vi "SimulatoreStep.vi"() -> ()   [LabVIEW 2019]
doc: "Simulatore Step dei Test:\n\n1. Seleziona la postazione con la data di partenza (opzionale)\n2. Seleziona il Test che vuoi eseguire\n3. Avvia la simulazione e verifica il successo degli Step"
uses:
  ByteGSAPIBase.lvclass
  TypeDef/StepSimulationInfo.ctl
  TypeDef/ProcessStatus.ctl
  TypeDef/SimulatoreStates.ctl
  TypeDef/Step.ctl
  TypeDef/Asset.ctl
  TypeDef/Test.ctl
  <vilib>/numeric/Random Number (Range) U64.vi
  <vilib>/numeric/sub_Random U32.vi
panel:
  out "Status Control":T2={"Cluster"={"Active"=FALSE, "Process"="Acquisizione Dati"}, "Cluster 2"={"Active"=FALSE, "Process"="Upload Dati"}, "Cluster 3"={"Active"=FALSE, "Process"="Upload Completato"}}
  out "Waveform Chart":cluster{"Time Elapsed":dbl, dbl}(graph)
  out "Step Info List":T3[](array[typedef])=[{"info"="Descrizione:\nMeasure T0\nMIN - MAX: 23 - 18", "Value"=0.0, "Outcome"="", "Tempo"=0.0, "id"=0.0}, {"info"="Descrizione:\nSet Nominsl Torque\nMIN - MAX: 1 - -1", "Value"=0.0, "Outcome"="", "Tempo"=0.0, "id"=0.0}, {"info"="Descrizione:\nVibrazione X,Y,Z\nMIN - MAX: 0 - 0", "Value"=0.0, "Outcome"="", "Tempo"=0.0, "id"=0.0}, {"info"="Descrizione:\nPlace Motor on the bench. Plug wires on terminal block.\nMIN - MAX: 0 - 0", "Value"=0.0, "Outcome"="", "Tempo"=0.0, "id"=0.0}, {"info"="Descrizione:\nMeasure R01\nMIN - MAX: 0 - 0", "Value"=0.0, "Outcome"="", "Tempo"=0.0, "id"=0.0}, {"info"="Descrizione:\nMeasure R02\nMIN - MAX: 0 - 0", "Value"=0.0, "Outcome"="", "Tempo"=0.0, "id"=0.0}]
  in  "Step simulation":bool
  out "Infos":string
  in  "Inizia Test":bool
  in  "Seleziona Test":i32(ring) items=["Test Endurance"=36, "Test su Statore H100 dia 65"=31, "Test su Statore H100 dia 65"=29, "Test Endurance"=34, "Test su Statore H100 dia 65"=30, "Effettuare prova sul banco Labview su campione ABC"=40, "Test su Statore H100 dia 65"=28, "Test su Statore H100 dia 65"=32, "Richiesta prova 1"=7, "Test Endurance"=35, "Richiesta prova 1"=5, "Richiesta prova 1"=6, "Test su Statore H100 dia 65"=27, "Test doppio carico per freni 50Nm/12rpm"=24]
  in  "ByteGSAPIBase in":refnum<class "ByteGSAPIBase.lvclass">
  in  "Exit":bool
  in  "Home":bool
  in  "Ottieni Test Per Postazione":bool
  in  "Data Partenza":timestamp format="%<%x>T"
  in  "Postazione":enum16{"POST 1"}(ring)
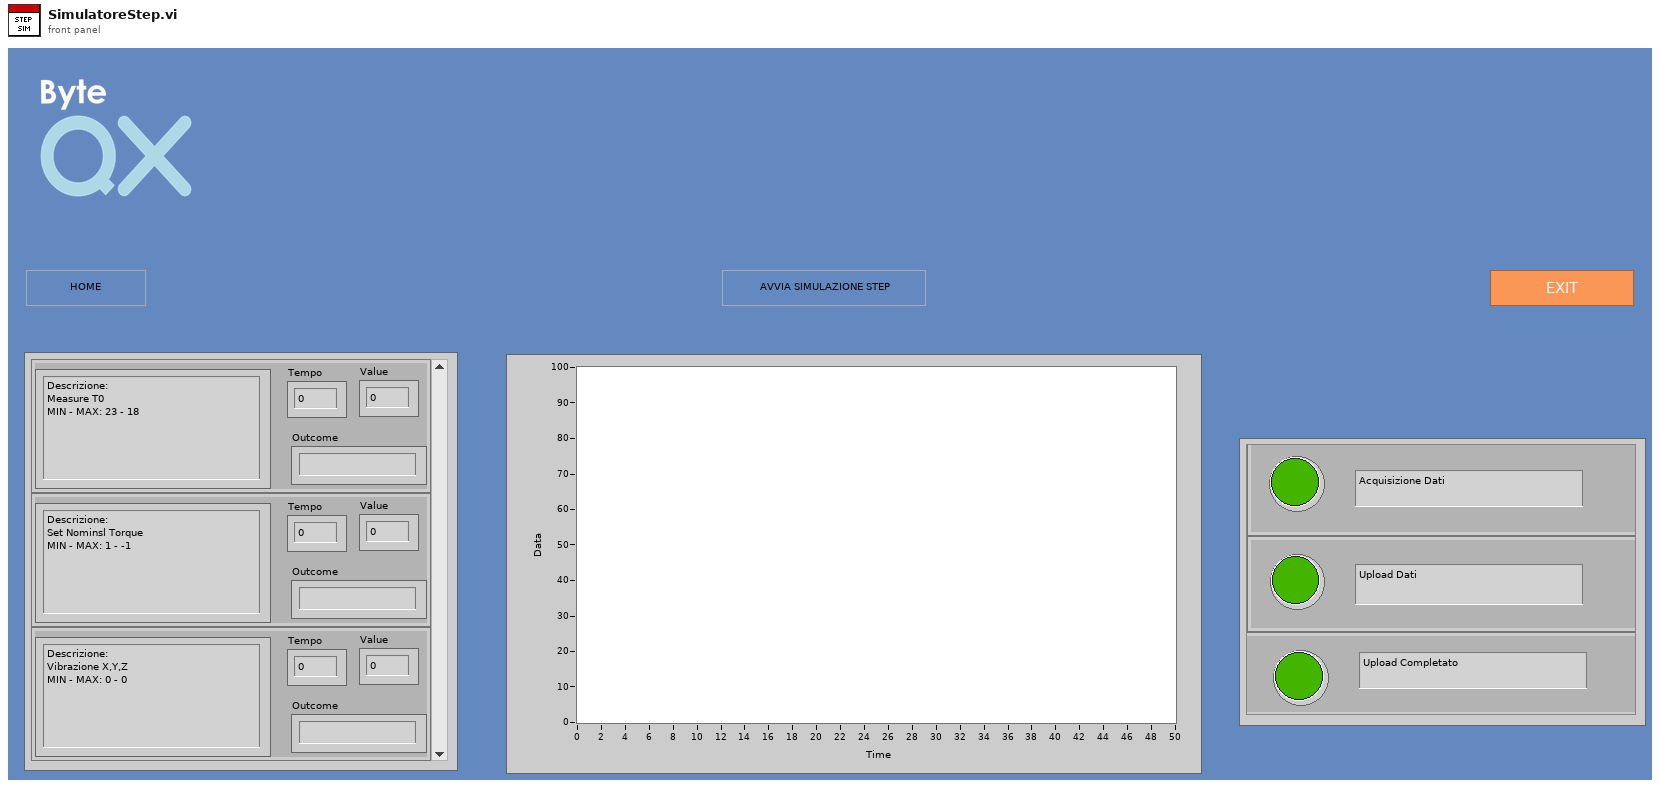
[diagram p1: front panel]
types:
  T1 = typedef "ProcessStatus.ctl" = cluster{"Active":bool, "Process":string}
  T2 = cluster{"Cluster":T1, "Cluster 2":T1, "Cluster 3":T1}
  T3 = typedef "StepSimulationInfo.ctl" = cluster{"info":string, "Value":dbl, "Outcome":string, "Tempo":dbl, "id":dbl}
  T4 = typedef "SimulatoreStates.ctl" = enum16{"Initialize", "Idle", "GetLimsTestsForBench", "GetLimsTestSteps", "Simulation Start", "WaitForLigths"}
  T5 = typedef "ByteGSWebAPI.lvlib/ByteGSAPIBase.lvclass/Test.ctl" = cluster{"titolo":string, "descrizione":string, "statoprova":string, "assets":T6[], "id":i32, "data_apertura_prova":timestamp}
  T6 = typedef "ByteGSWebAPI.lvlib/ByteGSAPIBase.lvclass/Asset.ctl" = cluster{"descrizione":string, "slug":string, "id":i32}
  T7 = typedef "ByteGSWebAPI.lvlib/ByteGSAPIBase.lvclass/Step.ctl" = cluster{"id":i32, "descrizione":string, "prova":string, "assets":T6[], "criterio_accettazione":string, "valore_criterio_accettazione_max":dbl, "valore_criterio_accettazione_min":dbl, "udm_criterio_accettazione":string, "duration_prova":string, "udm_duration_prova":string, "valore_prova":dbl, "ordine":i32, "user":i32, "link_automation":string, "instruction_automation":string, "data_completamento_checklist":timestamp, "outcome":bool}
  T8 = cluster{"ByteGSAPIBase in":refnum<class "ByteGSAPIBase.lvclass">, "Array dei Test":T5[], "Steps Array":T7[], "Step Info List":T3[], "index":i32, "Previus":T4, "Infos":string, "State":T4, "Status Control":cluster{"Cluster":T1, "Cluster 2":T1, "Cluster 3":T1}, "light position":i32}
  T9 = cluster{"Postazione":refnum<vi>, "Data Partenza":refnum<vi>, "Ottieni Test Per Postazione":refnum<vi>, "Infos":refnum<vi>, "Inizia Test":refnum<vi>, "Seleziona Test":refnum<vi>, "Step Info List":refnum<vi>, "Step simulation":refnum<vi>, "Cluster":refnum<vi>, "Waveform Chart":refnum<vi>, "Status Control":refnum<vi>}
  T10 = cluster{"Postazione":enum16{"POST 1"}, "Data Partenza":timestamp, "Seleziona Test":i32}
  T11 = typedef "ByteGSWebAPI.lvlib/ByteGSAPIBase.lvclass/UpdateLimsTestStepData.ctl" = cluster{"outcome":bool, "data_completamento_checklist":timestamp, "udm_duration_prova":string, "valore_prova":dbl, "link_automation":string, "instruction_automation":string, "duration_prova":string}
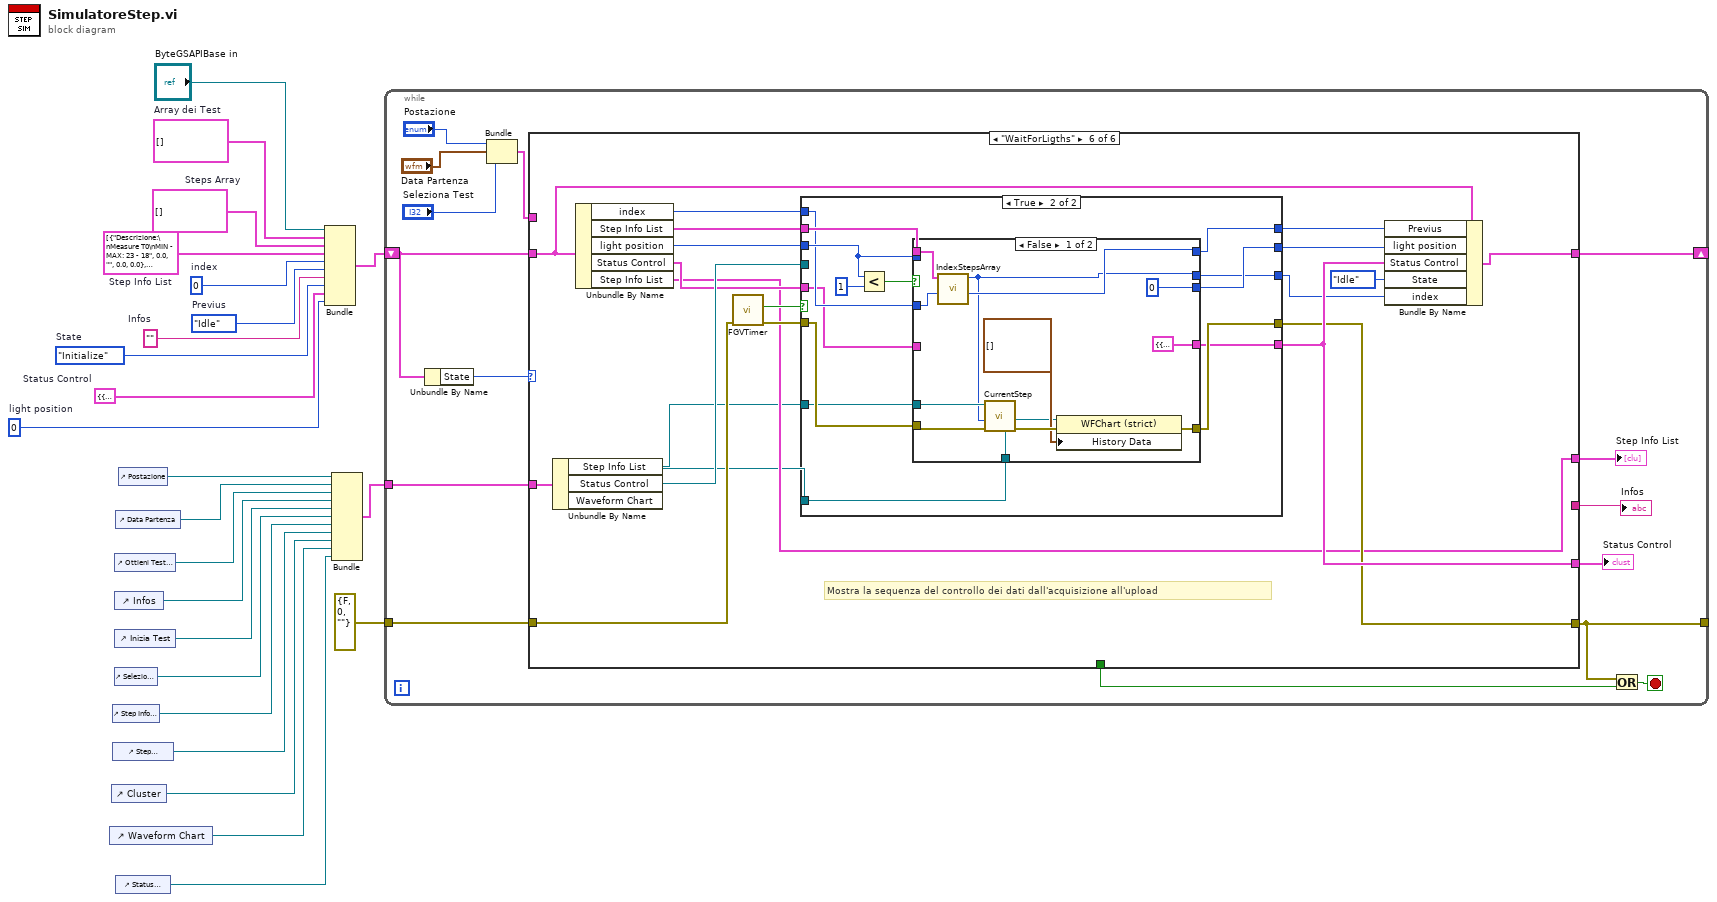
[diagram p0: block diagram]
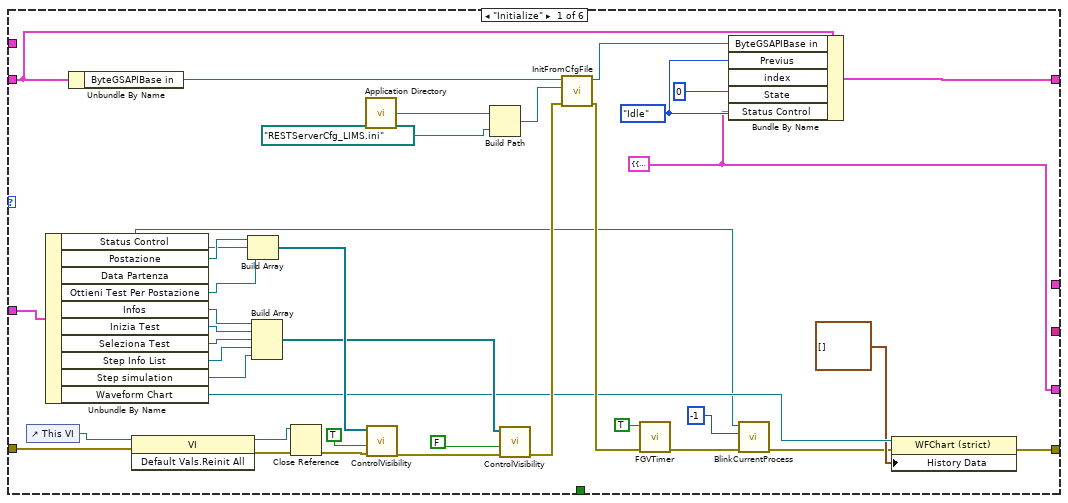
[diagram p2: hidden frame]
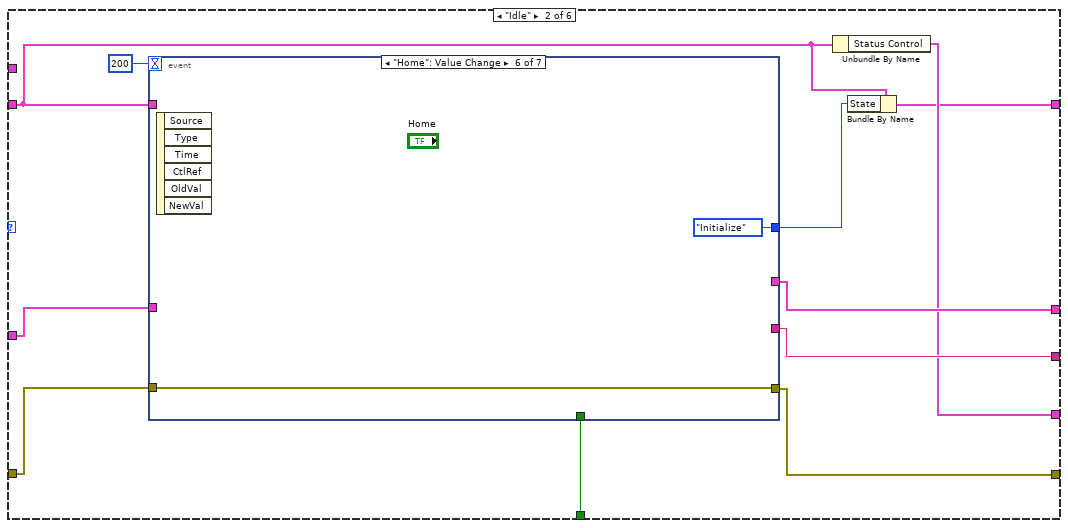
[diagram p3: hidden frame]
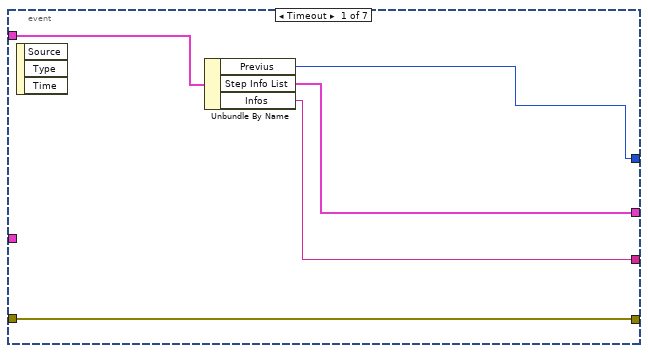
[diagram p4: hidden frame]
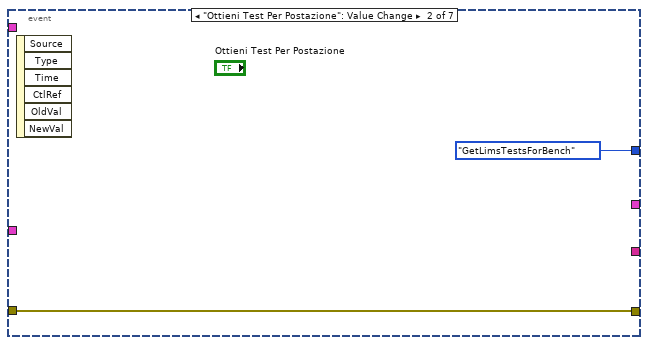
[diagram p5: hidden frame]
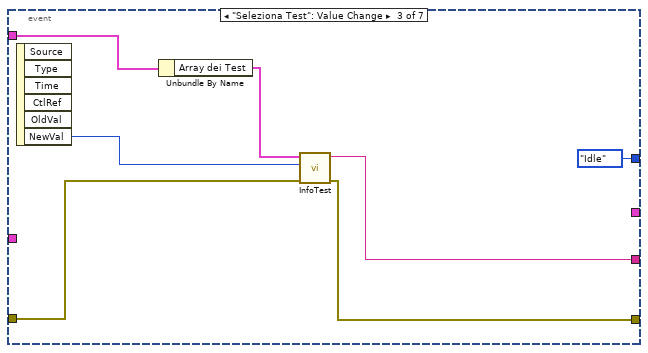
[diagram p6: hidden frame]
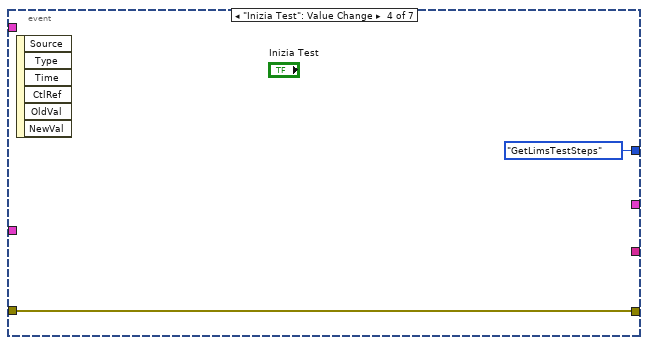
[diagram p7: hidden frame]
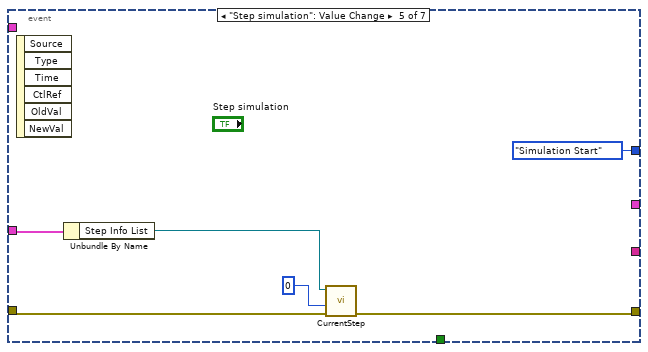
[diagram p8: hidden frame]
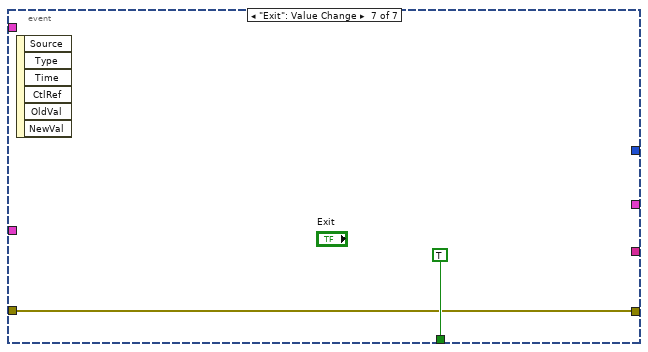
[diagram p9: hidden frame]
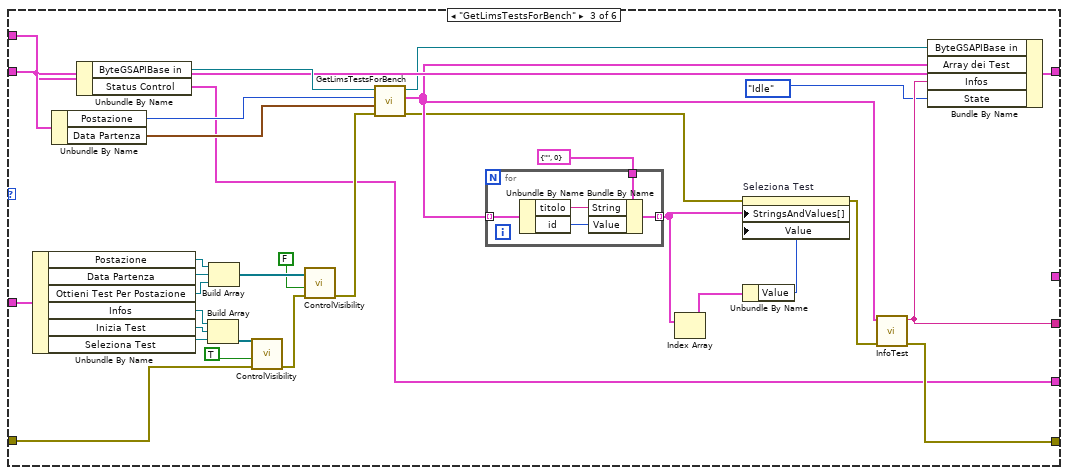
[diagram p10: hidden frame]
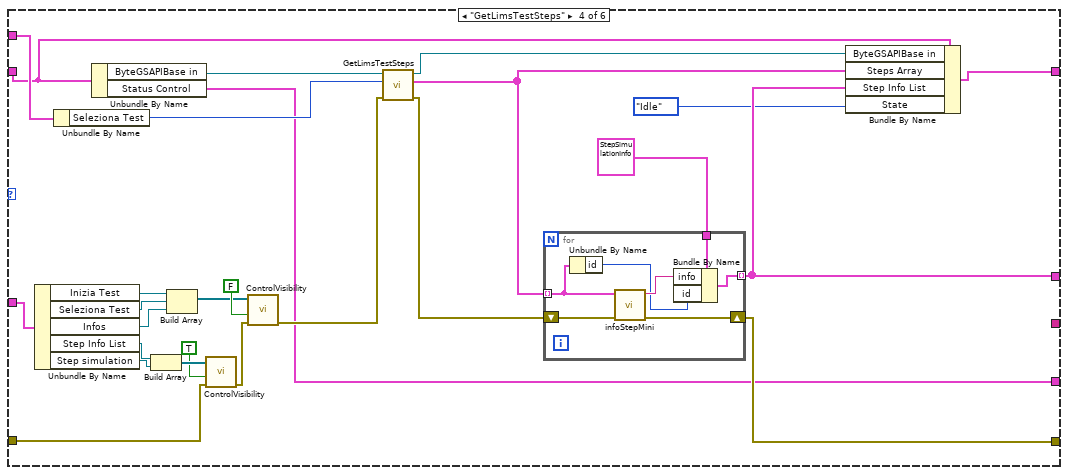
[diagram p11: hidden frame]
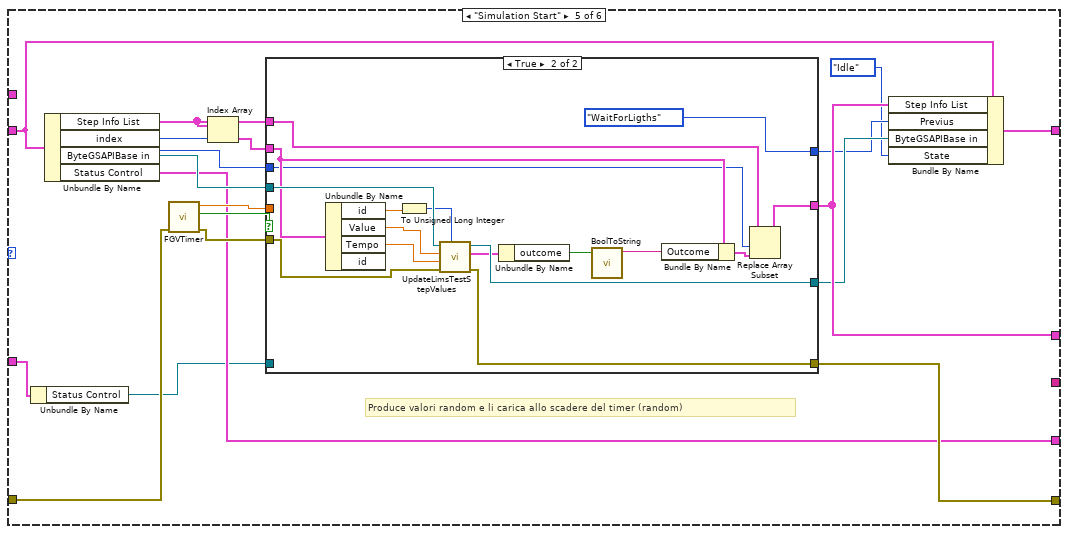
[diagram p12: hidden frame]
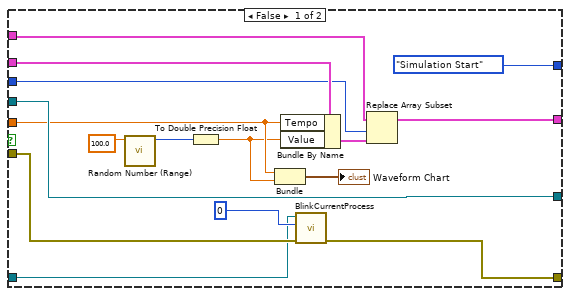
[diagram p13: hidden frame]
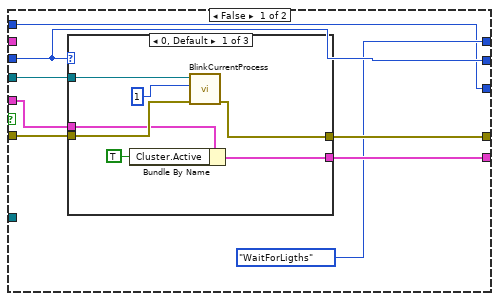
[diagram p14: hidden frame]
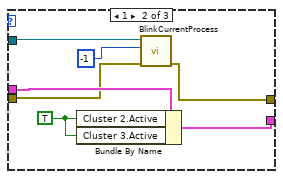
[diagram p15: hidden frame]
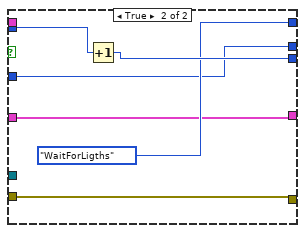
[diagram p17: hidden frame]
diagram:
  w1 = 0  # light position
  w2 = T2 {"Cluster"={"Active"=FALSE, "Process"="Acquisizione Dati"}, "Cluster 2"={"Active"=FALSE, "Process"="Upload Dati"}, "Cluster 3"={"Active"=FALSE, "Process"="Upload Completato"}}  # Status Control
  w9 = ""  # Infos
  w10 = SimulatoreStates."Idle"  # Previus
  w11 = 0  # index
  w12 = T3[] [{"info"="Descrizione:\nMeasure T0\nMIN - MAX: 23 - 18", "Value"=0.0, "Outcome"="", "Tempo"=0.0, "id"=0.0}, {"info"="Descrizione:\nSet Nominsl Torque\nMIN - MAX: 1 - -1", "Value"=0.0, "Outcome"="", "Tempo"=0.0, "id"=0.0}, {"info"="Descrizione:\nVibrazione X,Y,Z\nMIN - MAX: 0 - 0", "Value"=0.0, "Outcome"="", "Tempo"=0.0, "id"=0.0}, {"info"="Descrizione:\nPlace Motor on the bench. Plug wires on terminal block.\nMIN - MAX: 0 - 0", "Value"=0.0, "Outcome"="", "Tempo"=0.0, "id"=0.0}, {"info"="Descrizione:\nMeasure R01\nMIN - MAX: 0 - 0", "Value"=0.0, "Outcome"="", "Tempo"=0.0, "id"=0.0}, {"info"="Descrizione:\nMeasure R02\nMIN - MAX: 0 - 0", "Value"=0.0, "Outcome"="", "Tempo"=0.0, "id"=0.0}]  # Step Info List
  w19 = T5[] []  # Array dei Test
  w18 = T7[] []  # Steps Array
  w6 = SimulatoreStates."Initialize"  # State
  n1 = control-ref of="Waveform Chart"() -> (w5:refnum<vi>)
  n2 = control-ref of="Cluster"() -> (w7:refnum<vi>)
  n3 = control-ref of="Step Info List"() -> (w8:refnum<vi>)
  n4 = control-ref of="Step simulation"() -> (w13:refnum<vi>)
  n5 = control-ref of="Ottieni Test Per Postazione"() -> (w22:refnum<vi>)
  n6 = control-ref of="Infos"() -> (w16:refnum<vi>)
  n7 = control-ref of="Inizia Test"() -> (w15:refnum<vi>)
  n8 = control-ref of="Seleziona Test"() -> (w14:refnum<vi>)
  n9 = control-ref of="Data Partenza"() -> (w23:refnum<vi>)
  n10 = control-ref of="Status Control"() -> (w4:refnum<vi>)
  n11 = control-ref of="Postazione"() -> (w24:refnum<vi>)
  n12 = Bundle("ByteGSAPIBase in"="ByteGSAPIBase in", "Array dei Test"=w19, "Steps Array"=w18, "Step Info List"=w12, "index"=w11, "Previus"=w10, "Infos"=w9, "State"=w6, "Status Control"=w2, "light position"=w1) -> (w17:T8)  [unwired: 1 in]
  n13 = Bundle("Postazione"=w24, "Data Partenza"=w23, "Ottieni Test Per Postazione"=w22, "Infos"=w16, "Inizia Test"=w15, "Seleziona Test"=w14, "Step Info List"=w8, "Step simulation"=w13, "Cluster"=w7, "Waveform Chart"=w5, "Status Control"=w4) -> (w21:T9)  [unwired: 1 in]
  n14 = while {
    tunnel: w21 -> [w35]
    shift-right: [w34] -> _
    shift-left: w17 -> [w27]
    tunnel: errorcluster {"status"=FALSE, "code"=0, "source"=""} ("error in (no error)") -> [w39]
    tunnel: [w30] -> _
    stop <- w29 stop-if-true
    n15 = Unbundle By Name(w27) -> ("State"=w26:T4)
    n16 = Bundle("Postazione"="Postazione", "Data Partenza"="Data Partenza", "Seleziona Test"="Seleziona Test") -> (w36:T10)  [unwired: 1 in]
    n17 = case shown="\"WaitForLigths\"" w26 {
      tunnel: w39 -> [w77 w89 w141 w160 w202 w252]
      tunnel: w36 -> [_ _ w146 w178 _ _]
      tunnel: w35 -> [w74 w83 w136 w172 w189 w254]
      tunnel: [w47 w87 w125 w165 w191 w245] -> w30
      tunnel: w27 -> [w62 w80 w145 w175 w199 w249]
      tunnel: [w61 w79 w143 w174 w195 w248] -> w34
      tunnel: [_ w88 w120 _ _ _] -> w32
      tunnel: [_ w85 _ w156 w196 w242] -> w31
      tunnel: [_ w84 _ _ _ _] -> w28
      tunnel: [w40 w81 w116 w153 w187 w246] -> w25
      frame "Initialize" {
        w40 = T2 {"Cluster"={"Active"=FALSE, "Process"="Acquisizione Dati"}, "Cluster 2"={"Active"=FALSE, "Process"="Upload Dati"}, "Cluster 3"={"Active"=FALSE, "Process"="Upload Completato"}} ("Status Control")
        w48 = SimulatoreStates."Idle"
        n18 = control-ref of="This VI"() -> (w78:refnum<vi>)
        n19 = Unbundle By Name(w74) -> ("Status Control"=w41:refnum<vi>, "Postazione"=w73:refnum<vi>, "Data Partenza"=w72:refnum<vi>, "Ottieni Test Per Postazione"=w71:refnum<vi>, "Infos"=w57:refnum<vi>, "Inizia Test"=w56:refnum<vi>, "Seleziona Test"=w55:refnum<vi>, "Step Info List"=w53:refnum<vi>, "Step simulation"=w52:refnum<vi>, "Waveform Chart"=w46:refnum<vi>)
        n20 = Unbundle By Name(w62) -> ("ByteGSAPIBase in"=w63:refnum<class "ByteGSAPIBase.lvclass">)
        n21 = invoke class="VI" method="Default Vals.Reinit All"(reference=w78, error in=w77) -> (reference out=w76:refnum<vi>, error out=w75:errorcluster)  [unwired: 1 in, 1 out]
        n22 = Build Array(w73, w72, w71) -> (w70:refnum<vi>[])
        n23 = Build Array(w57, w56, w55, w53, w52) -> (w54:refnum<vi>[])
        n24 = Close Reference(reference=w76, error in (no error)=w75) -> (error out=w69:errorcluster)
        n25 = call <vilib>:"Application Directory.vi"() -> ("Application Directory"=w66:path)
        n26 = call "ControlVisibility.vi"("error in (no error)"=w69, "Visible"=TRUE, "Controls"=w70) -> ("error out"=w60:errorcluster)  [unwired: 8 in]
        n27 = Build Path(base path=w66, name or relative path=path "RESTServerCfg_LIMS.ini") -> (appended path=w67:path)
        n28 = call "ControlVisibility.vi"("error in (no error)"=w60, "Visible"=FALSE, "Controls"=w54) -> ("error out"=w59:errorcluster)  [unwired: 8 in]
        n29 = call-dynamic "InitFromCfgFile.vi"("error in (no error)"=w59, "configuration file path"=w67, "ByteGSAPIBase in"=w63) -> ("error out"=w51:errorcluster, "ByteGSAPIBase out"=w64:refnum<class "ByteGSAPIBase.lvclass">)  [unwired: 7 in]
        n30 = call "FGVTimer.vi"("error in"=w51, "Reset"=TRUE) -> ("error out"=w44:errorcluster)  [unwired: 7 in, 2 out]
        n31 = Bundle By Name(cluster=w62, "ByteGSAPIBase in"=w64, "Previus"=w48, "index"=0, "State"=w48, "Status Control"=w40) -> (w61:T8)
        n32 = call "BlinkCurrentProcess.vi"("error in (no error)"=w44, "index"=-1, "Status Control"=w41) -> ("error out"=w43:errorcluster)  [unwired: 8 in]
        n33 = property class="WFChart (strict)"(reference=w46, error in=w43, "History Data"=cluster{"Time Elapsed":dbl, dbl}[] []) -> (error out=w47:errorcluster)  [unwired: 1 out]
      }
      frame "Idle" {
        n34 = event shown="[5] \"Home\": Value Change" {
          selector: _ -> [_ _ _ _ _ _ _]
          dyn-events: _ -> [_ _ _ _ _ _ _]
          timeout: 200 -> [_ _ _ _ _ _ _]
          tunnel: [w90 SimulatoreStates."GetLimsTestsForBench" SimulatoreStates."Idle" SimulatoreStates."GetLimsTestSteps" SimulatoreStates."Simulation Start" SimulatoreStates."Initialize" _] -> w82
          tunnel: [w92 _ w101 _ _ _ _] -> w88
          tunnel: w89 -> [w91 w95 w100 w104 w109 w112 w114]
          tunnel: [w91 w95 w99 w104 w108 w112 w114] -> w87
          tunnel: w80 -> [w94 _ w98 _ _ _ _]
          tunnel: [w93 _ _ _ _ _ _] -> w85
          tunnel: [_ _ _ _ _ _ TRUE] -> w84
          tunnel: w83 -> [_ _ _ _ w110 _ _]
          event Timeout {
            n35 = event-data() -> ()  [unwired: 1 in, 3 out]
            n36 = Unbundle By Name(w94) -> ("Previus"=w90:T4, "Step Info List"=w93:T3[], "Infos"=w92:string)
          }
          event "Ottieni Test Per Postazione": Value Change {
            n37 = event-data() -> ()  [unwired: 1 in, 6 out]
          }
          event "Seleziona Test": Value Change {
            n38 = event-data() -> ("NewVal"=w97:i32)  [unwired: 1 in, 5 out]
            n39 = Unbundle By Name(w98) -> ("Array dei Test"=w102:T5[])
            n40 = call "InfoTest.vi"("error in"=w100, "Seleziona Test"=w97, "TestForBenchArray"=w102) -> ("error out"=w99:errorcluster, "Info Test"=w101:string)  [unwired: 7 in]
          }
          event "Inizia Test": Value Change {
            n41 = event-data() -> ()  [unwired: 1 in, 6 out]
          }
          event "Step simulation": Value Change {
            n42 = event-data() -> ()  [unwired: 1 in, 6 out]
            n43 = Unbundle By Name(w110) -> ("Step Info List"=w107:refnum<vi>)
            n44 = call "CurrentStep.vi"("error in (no error)"=w109, "index"=0, "Array in"=w107) -> ("error out"=w108:errorcluster)  [unwired: 8 in]
          }
          event "Home": Value Change {
            n45 = event-data() -> ()  [unwired: 1 in, 6 out]
          }
          event "Exit": Value Change {
            n46 = event-data() -> ()  [unwired: 1 in, 6 out]
          }
        }
        n47 = Unbundle By Name(w80) -> ("Status Control"=w81:T2)
        n48 = Bundle By Name(cluster=w80, "State"=w82) -> (w79:T8)
      }
      frame "GetLimsTestsForBench" {
        n49 = Unbundle By Name(w136) -> ("Postazione"=w135:refnum<vi>, "Data Partenza"=w134:refnum<vi>, "Ottieni Test Per Postazione"=w133:refnum<vi>, "Infos"=w132:refnum<vi>, "Inizia Test"=w131:refnum<vi>, "Seleziona Test"=w130:refnum<vi>)
        n50 = Unbundle By Name(w146) -> ("Postazione"=w119:enum16{"POST 1"}, "Data Partenza"=w118:timestamp)
        n51 = Unbundle By Name(w145) -> ("ByteGSAPIBase in"=w147:refnum<class "ByteGSAPIBase.lvclass">, "Status Control"=w116:T2)
        n52 = Build Array(w132, w131, w130) -> (w123:refnum<vi>[])
        n53 = Build Array(w135, w134, w133) -> (w124:refnum<vi>[])
        n54 = call "ControlVisibility.vi"("error in (no error)"=w141, "Visible"=TRUE, "Controls"=w123) -> ("error out"=w129:errorcluster)  [unwired: 8 in]
        n55 = call "ControlVisibility.vi"("error in (no error)"=w129, "Visible"=FALSE, "Controls"=w124) -> ("error out"=w128:errorcluster)  [unwired: 8 in]
        n56 = call-dynamic "GetLimsTestsForBench.vi"("error in (no error)"=w128, "Data Partenza"=w118, "Postazione"=w119, "ByteGSAPIBase in"=w147) -> ("error out"=w127:errorcluster, "Tests for bench"=w137:T5[], "ByteGSAPIBase out"=w144:refnum<class "ByteGSAPIBase.lvclass">)  [unwired: 5 in]
        n57 = for {
          tunnel: w137 -> [w152] mode=indexing
          tunnel: [w149] -> w140 mode=indexing
          tunnel: cluster{"String":string, "Value":u16} {"String"="", "Value"=0} ("Cluster") -> [w148]
          n58 = Unbundle By Name(w152) -> ("titolo"=w151:string, "id"=w150:i32)
          n59 = Bundle By Name(cluster=w148, "String"=w151, "Value"=w150) -> (w149:cluster{"String":string, "Value":u16})
        }
        n60 = Index Array(array=w140) -> (element=w139:cluster{"String":string, "Value":u16})  [unwired: 1 in]
        n61 = Unbundle By Name(w139) -> ("Value"=w138:u16)
        n62 = property on="Seleziona Test" class="Ring (strict)"(error in=w127, "StringsAndValues[]"=w140, "Value"=w138) -> (error out=w126:errorcluster)  [unwired: 1 in, 1 out]
        n63 = call "InfoTest.vi"("error in"=w126, "TestForBenchArray"=w137) -> ("error out"=w125:errorcluster, "Info Test"=w120:string)  [unwired: 8 in]
        n64 = Bundle By Name(cluster=w145, "ByteGSAPIBase in"=w144, "Array dei Test"=w137, "Infos"=w120, "State"=SimulatoreStates."Idle") -> (w143:T8)
      }
      frame "GetLimsTestSteps" {
        n65 = Unbundle By Name(w172) -> ("Inizia Test"=w171:refnum<vi>, "Seleziona Test"=w170:refnum<vi>, "Infos"=w163:refnum<vi>, "Step Info List"=w162:refnum<vi>, "Step simulation"=w157:refnum<vi>)
        n66 = Unbundle By Name(w178) -> ("Seleziona Test"=w164:i32)
        n67 = Unbundle By Name(w175) -> ("ByteGSAPIBase in"=w177:refnum<class "ByteGSAPIBase.lvclass">, "Status Control"=w153:T2)
        n68 = Build Array(w162, w157) -> (w161:refnum<vi>[])
        n69 = Build Array(w171, w170, w163) -> (w169:refnum<vi>[])
        n70 = call "ControlVisibility.vi"("error in (no error)"=w160, "Visible"=TRUE, "Controls"=w161) -> ("error out"=w159:errorcluster)  [unwired: 8 in]
        n71 = call "ControlVisibility.vi"("error in (no error)"=w159, "Visible"=FALSE, "Controls"=w169) -> ("error out"=w168:errorcluster)  [unwired: 8 in]
        n72 = call-dynamic "GetLimsTestSteps.vi"("error in (no error)"=w168, "Test-id"=w164, "ByteGSAPIBase in"=w177) -> ("error out"=w166:errorcluster, "Test Steps List"=w167:T7[], "ByteGSAPIBase out"=w176:refnum<class "ByteGSAPIBase.lvclass">)  [unwired: 6 in]
        n73 = for {
          tunnel: w167 -> [w180] mode=indexing
          shift-right: [w184] -> w165
          shift-left: w166 -> [w185]
          tunnel: T3 {"info"="Descrizione:\nMeasure T0\nMIN - MAX: 23 - 18", "Value"=0.0, "Outcome"="", "Tempo"=0.0, "id"=0.0} ("Cluster") -> [w183]
          tunnel: [w181] -> w156 mode=indexing
          n74 = Unbundle By Name(w180) -> ("id"=w179:i32)
          n75 = call "infoStepMini.vi"("error in (no error)"=w185, "StepList"=w180) -> ("error out"=w184:errorcluster, "Info Test"=w182:string)  [unwired: 8 in]
          n76 = Bundle By Name(cluster=w183, "info"=w182, "id"=w179) -> (w181:T3)
        }
        n77 = Bundle By Name(cluster=w175, "ByteGSAPIBase in"=w176, "Steps Array"=w167, "Step Info List"=w156, "State"=SimulatoreStates."Idle") -> (w174:T8)
      }
      frame "Simulation Start" {
        # "Produce valori random e li carica allo scadere del timer (random)"
        n78 = Unbundle By Name(w189) -> ("Status Control"=w186:refnum<vi>)
        n79 = Unbundle By Name(w199) -> ("Step Info List"=w198:T3[], "index"=w197:i32, "ByteGSAPIBase in"=w194:refnum<class "ByteGSAPIBase.lvclass">, "Status Control"=w187:T2)
        n80 = call "FGVTimer.vi"("error in"=w202) -> ("error out"=w193:errorcluster, "Elapsed?"=w203:bool, "Time Elapsed"=w200:dbl)  [unwired: 8 in]
        n81 = Index Array(array=w198, index=w197) -> (element=w201:T3)
        n82 = case shown="True" w203 {
          tunnel: w201 -> [w219 w233]
          tunnel: w200 -> [w209 _]
          tunnel: w198 -> [w217 w227]
          tunnel: w197 -> [w211 w228]
          tunnel: [w215 w236] -> w196
          tunnel: w194 -> [w214 w234]
          tunnel: w193 -> [w207 w224]
          tunnel: [w214 w230] -> w192
          tunnel: [w206 w222] -> w191
          tunnel: [SimulatoreStates."Simulation Start" ("Previus") SimulatoreStates."WaitForLigths" ("Previus")] -> w190
          tunnel: w186 -> [w204 _]
          frame False {
            n83 = call-poly <vilib>:"Random Number (Range).vi"("upper bound (100)"=100.0) -> ("number"=w212:u64)  [unwired: 10 in]
            n84 = To Double Precision Float(number=w212) -> (double precision float=w208:dbl)
            n85 = Bundle("Time Elapsed"=w209, w208) -> (→"Waveform Chart":cluster{"Time Elapsed":dbl, dbl})  [unwired: 1 in]
            n86 = Bundle By Name(cluster=w219, "Tempo"=w209, "Value"=w208) -> (w216:T3)
            n87 = call "BlinkCurrentProcess.vi"("error in (no error)"=w207, "index"=0, "Status Control"=w204) -> ("error out"=w206:errorcluster)  [unwired: 8 in]
            n88 = Replace Array Subset(array=w217, new element=w216, index=w211) -> (w215:T3[])
          }
          frame True {
            n89 = Unbundle By Name(w233) -> ("id"=w221:dbl, "Value"=w232:dbl, "Tempo"=w231:dbl)  [unwired: 1 out]
            n90 = To Unsigned Long Integer(number=w221) -> (unsigned 32bit integer=w220:u32)
            n91 = call-dynamic "UpdateLimsTestStepValues.vi"("step_id"=w220, "error in (no error)"=w224, "duration_hours"=w231, "value"=w232, "ByteGSAPIBase in"=w234) -> ("error out"=w222:errorcluster, "Result Step"=w229:T11, "ByteGSAPIBase out"=w230:refnum<class "ByteGSAPIBase.lvclass">)  [unwired: 4 in]
            n92 = Unbundle By Name(w229) -> ("outcome"=w225:bool)
            n93 = call "BoolToString.vi"("outcome"=w225) -> ("String"=w226:string)  [unwired: 10 in]
            n94 = Bundle By Name(cluster=w233, "Outcome"=w226) -> (w235:T3)
            n95 = Replace Array Subset(array=w227, new element=w235, index=w228) -> (w236:T3[])
          }
        }
        n96 = Bundle By Name(cluster=w199, "Step Info List"=w196, "Previus"=w190, "ByteGSAPIBase in"=w192, "State"=SimulatoreStates."Idle") -> (w195:T8)
      }
      frame "WaitForLigths" {
        # "Mostra la sequenza del controllo dei dati dall'acquisizione all'upload"
        n97 = Unbundle By Name(w254) -> ("Step Info List"=w238:refnum<vi>, "Status Control"=w253:refnum<vi>, "Waveform Chart"=w237:refnum<vi>)
        n98 = Unbundle By Name(w249) -> ("index"=w240:i32, "Step Info List"=w241:T3[], "light position"=w255:i32, "Status Control"=w250:T2, "Step Info List"=w242:T3[])
        n99 = call "FGVTimer.vi"("error in"=w252) -> ("error out"=w251:errorcluster, "Elapsed?"=w256:bool)  [unwired: 8 in, 1 out]
        n100 = case shown="True" w256 {
          tunnel: w255 -> [w259 w292]
          tunnel: w253 -> [w264 _]
          tunnel: w251 -> [w263 w286]
          tunnel: w250 -> [w262 w281]
          tunnel: [w261 w282] -> w246
          tunnel: [w260 w284] -> w245
          tunnel: [w259 w291] -> w244
          tunnel: [SimulatoreStates."WaitForLigths" ("Previus") w290] -> w243
          tunnel: w241 -> [_ w289]
          tunnel: w240 -> [w257 w288]
          tunnel: [w257 w287] -> w239
          tunnel: w238 -> [_ w285]
          tunnel: w237 -> [_ w283]
          frame False {
            n101 = case shown="0, Default" w259 {
              tunnel: w264 -> [w270 w277 _]
              tunnel: w263 -> [w269 w275 w279]
              tunnel: w262 -> [w267 w276 w280]
              tunnel: [w266 w274 w280] -> w261
              tunnel: [w265 w273 w279] -> w260
              frame 0, Default {
                n102 = Bundle By Name(cluster=w267, "Cluster.Active"=TRUE) -> (w266:T2)
                n103 = call "BlinkCurrentProcess.vi"("error in (no error)"=w269, "index"=1, "Status Control"=w270) -> ("error out"=w265:errorcluster)  [unwired: 8 in]
              }
              frame 1 {
                w272 = TRUE ("Cluster.Active")
                n104 = Bundle By Name(cluster=w276, "Cluster 2.Active"=w272, "Cluster 3.Active"=w272) -> (w274:T2)
                n105 = call "BlinkCurrentProcess.vi"("error in (no error)"=w275, "index"=-1, "Status Control"=w277) -> ("error out"=w273:errorcluster)  [unwired: 8 in]
              }
              frame 2 {
              }
            }
          }
          frame True {
            n106 = Less?(x=w292, y=1) -> (x < y?=w293:bool)
            n107 = case shown="False" w293 {
              tunnel: w292 -> [_ w312]
              tunnel: [0 w311] -> w291
              tunnel: [w305 SimulatoreStates."WaitForLigths" ("Previus")] -> w290
              tunnel: w289 -> [w304 _]
              tunnel: w288 -> [w301 w309]
              tunnel: [w295 w309] -> w287
              tunnel: w286 -> [w303 w308]
              tunnel: w285 -> [w302 _]
              tunnel: [w298 w308] -> w284
              tunnel: w283 -> [w297 _]
              tunnel: [T2 {"Cluster"={"Active"=FALSE, "Process"="Acquisizione Dati"}, "Cluster 2"={"Active"=FALSE, "Process"="Upload Dati"}, "Cluster 3"={"Active"=FALSE, "Process"="Upload Completato"}} ("Status Control") w307] -> w282
              tunnel: w281 -> [_ w307]
              frame False {
                n108 = call "IndexStepsArray.vi"("index"=w301, "Steps Array"=w304) -> ("Previus"=w305:T4, "Index out"=w295:i32)  [unwired: 8 in]
                n109 = call "CurrentStep.vi"("error in (no error)"=w303, "index"=w295, "Array in"=w302) -> ("error out"=w300:errorcluster)  [unwired: 8 in]
                n110 = property class="WFChart (strict)"(reference=w297, error in=w300, "History Data"=cluster{"Time Elapsed":dbl, dbl}[] []) -> (error out=w298:errorcluster)  [unwired: 1 out]
              }
              frame True {
                n111 = Increment(x=w312) -> (x+1=w311:i32)
              }
            }
          }
        }
        n112 = Bundle By Name(cluster=w249, "Previus"=w243, "light position"=w244, "Status Control"=w246, "State"=SimulatoreStates."Idle", "index"=w239) -> (w248:T8)
      }
    }
    "Infos" <- w32
    "Step Info List" <- w31
    "Status Control" <- w25
    n113 = Or(x=w30, y=w28) -> (x .or. y?=w29:bool)
  }
